vi "ReadIOValues b2g1.vi"(2 "error in":errorcluster, 3 "Output - Cluster b2g1 2":T1 {"DS-3 [bar]" format="%#.2g"; "TS-6 [°C]" format="%#.2g"; "GZ-1 [dl]" format="%.0g"; "TS-5 [°C]" format="%#.2g"; "pHS-1 [pH]" format="%.2g"; "TS-4 [°C]" format="%#.2g"; "FS-2 [l]" format="%.2g"; "FS-1 [l]" format="%.2g"; "DS-1 [bar]" format="%#.2g"; "DFS-1 [l/min]" format="%#.2g"; "FS-3 [l]" format="%.2g"; "DFS-1 [dl]" format="%.0g"}) -> (0 "error out":errorcluster, 1 "Output - Cluster b2g1":T1 {"DS-3 [bar]" format="%#.2g"; "TS-6 [°C]" format="%#.2g"; "GZ-1 [dl]" format="%.0g"; "TS-5 [°C]" format="%#.2g"; "pHS-1 [pH]" format="%.2g"; "TS-4 [°C]" format="%#.2g"; "FS-2 [l]" format="%.2g"; "FS-1 [l]" format="%.2g"; "DS-1 [bar]" format="%#.2g"; "DFS-1 [l/min]" format="%#.2g"; "FS-3 [l]" format="%.2g"; "DFS-1 [dl]" format="%.0g"})   [LabVIEW 2011]
uses:
  <vilib>/functionblocks/Counter/Count Up/Count Up.vi
  <vilib>/functionblocks/NI_FunctionBlock Libraries.lvlib
  <vilib>/functionblocks/FB Core/FB Core.xnode
  Output - Cluster b2g1.ctl
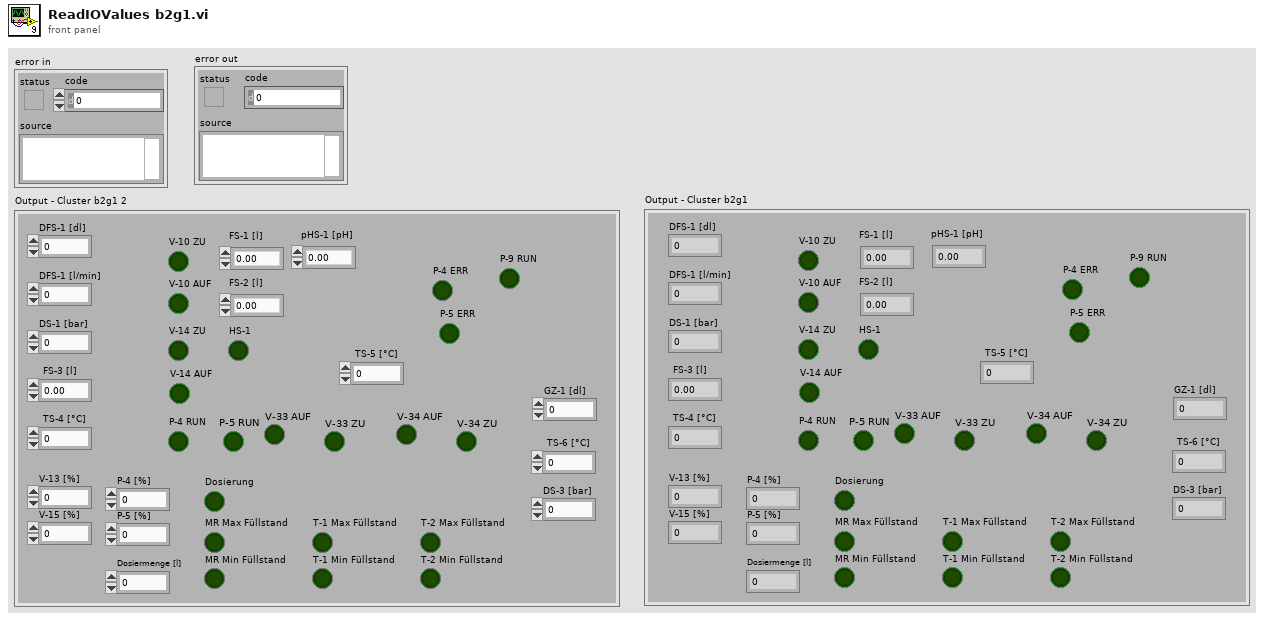
[diagram p1: front panel]
types:
  T1 = typedef "Output - Cluster b2g1.ctl" = cluster{"DFS-1 [dl]":u64, "FS-3 [l]":dbl, "DFS-1 [l/min]":dbl, "DS-1 [bar]":dbl, "V-10 ZU":bool, "V-14 ZU":bool, "FS-1 [l]":dbl, "FS-2 [l]":dbl, "TS-4 [°C]":dbl, "HS-1":bool, "V-13 [%]":u8, "V-15 [%]":u8, "P-4 [%]":u8, "P-5 [%]":u8, "Dosierung":bool, "MR Max Füllstand":bool, "MR Min Füllstand":bool, "Dosiermenge [l]":sgl, "V-14 AUF":bool, "V-10 AUF":bool, "T-1 Max Füllstand":bool, "T-1 Min Füllstand":bool, "T-2 Max Füllstand":bool, "T-2 Min Füllstand":bool, "pHS-1 [pH]":dbl, "P-4 RUN":bool, "P-5 RUN ":bool, "V-33 AUF":bool, "V-33 ZU":bool, "V-34 AUF":bool, "V-34 ZU":bool, "P-4 ERR":bool, "P-5 ERR":bool, "TS-5 [°C]":dbl, "GZ-1 [dl]":u64, "TS-6 [°C]":dbl, "DS-3 [bar]":dbl, "P-9 RUN":bool}
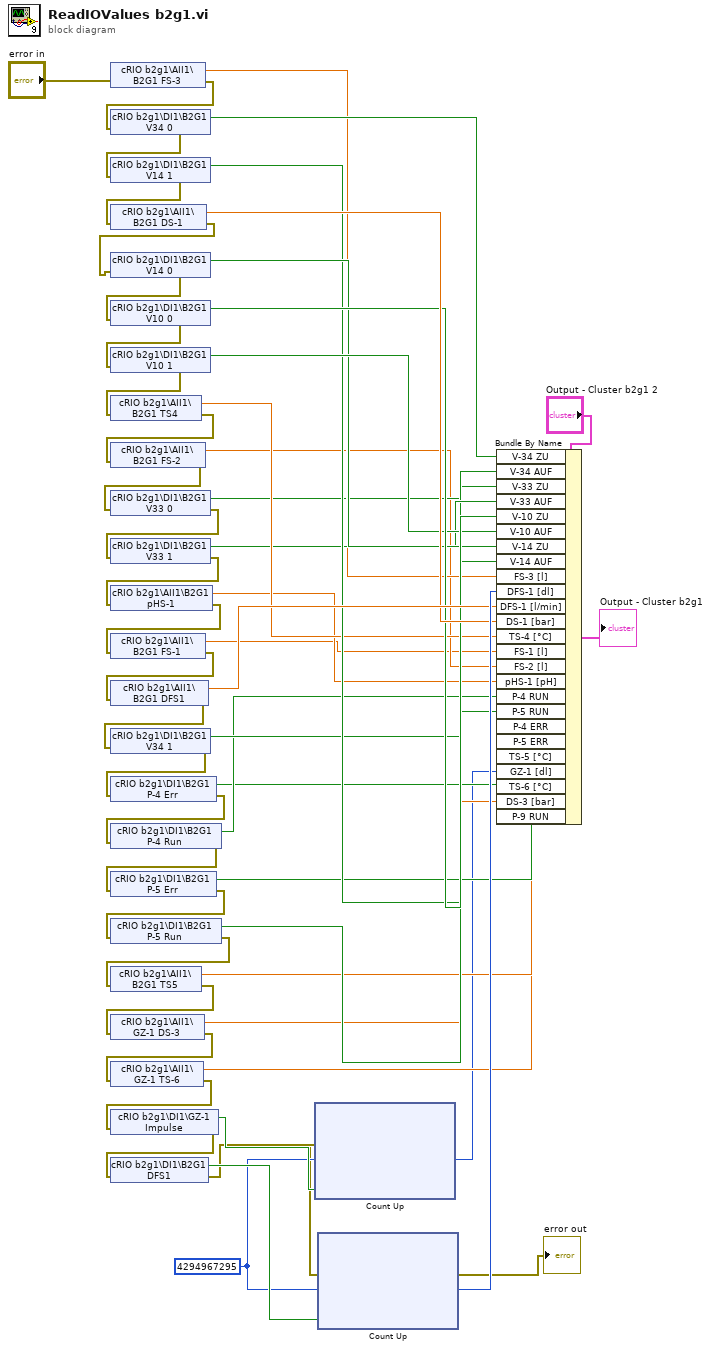
[diagram p0: block diagram]
diagram:
  w37 = u32 4294967295 ("preset value")
  n1 = shared-variable "cRIO b2g1\\AII1\\B2G1 FS-3"(error in="error in") -> (w19:dbl, error out=w26:errorcluster)
  n2 = shared-variable "cRIO b2g1\\DI1\\B2G1 V34 0"(error in=w26) -> (w45:bool, error out=w25:errorcluster)
  n3 = shared-variable "cRIO b2g1\\DI1\\B2G1 V14 1"(error in=w25) -> (w49:bool, error out=w24:errorcluster)
  n4 = shared-variable "cRIO b2g1\\AII1\\B2G1 DS-1"(error in=w24) -> (w53:dbl, error out=w23:errorcluster)
  n5 = shared-variable "cRIO b2g1\\DI1\\B2G1 V14 0"(error in=w23) -> (w50:bool, error out=w22:errorcluster)
  n6 = shared-variable "cRIO b2g1\\DI1\\B2G1 V10 0"(error in=w22) -> (w52:bool, error out=w21:errorcluster)
  n7 = shared-variable "cRIO b2g1\\DI1\\B2G1 V10 1"(error in=w21) -> (w51:bool, error out=w20:errorcluster)
  n8 = shared-variable "cRIO b2g1\\AII1\\B2G1 TS4"(error in=w20) -> (w48:dbl, error out=w17:errorcluster)
  n9 = shared-variable "cRIO b2g1\\AII1\\B2G1 FS-2"(error in=w17) -> (w2:dbl, error out=w16:errorcluster)
  n10 = shared-variable "cRIO b2g1\\DI1\\B2G1 V33 0"(error in=w16) -> (w18:bool, error out=w15:errorcluster)
  n11 = shared-variable "cRIO b2g1\\DI1\\B2G1 V33 1"(error in=w15) -> (w46:bool, error out=w14:errorcluster)
  n12 = shared-variable "cRIO b2g1\\AII1\\B2G1 pHS-1"(error in=w14) -> (w47:dbl, error out=w13:errorcluster)
  n13 = shared-variable "cRIO b2g1\\AII1\\B2G1 FS-1"(error in=w13) -> (w1:dbl, error out=w12:errorcluster)
  n14 = shared-variable "cRIO b2g1\\AII1\\B2G1 DFS1"(error in=w12) -> (w54:dbl, error out=w11:errorcluster)
  n15 = shared-variable "cRIO b2g1\\DI1\\B2G1 V34 1"(error in=w11) -> (w44:bool, error out=w10:errorcluster)
  n16 = shared-variable "cRIO b2g1\\DI1\\B2G1 P-4 Err"(error in=w10) -> (w41:bool, error out=w9:errorcluster)
  n17 = shared-variable "cRIO b2g1\\DI1\\B2G1 P-4 Run"(error in=w9) -> (w43:bool, error out=w8:errorcluster)
  n18 = shared-variable "cRIO b2g1\\DI1\\B2G1 P-5 Err"(error in=w8) -> (w40:bool, error out=w7:errorcluster)
  n19 = shared-variable "cRIO b2g1\\DI1\\B2G1 P-5 Run"(error in=w7) -> (w42:bool, error out=w6:errorcluster)
  n20 = shared-variable "cRIO b2g1\\AII1\\B2G1 TS5"(error in=w6) -> (w39:dbl, error out=w3:errorcluster)
  n21 = shared-variable "cRIO b2g1\\AII1\\GZ-1 DS-3"(error in=w3) -> (w35:dbl, error out=w5:errorcluster)
  n22 = shared-variable "cRIO b2g1\\AII1\\GZ-1 TS-6"(error in=w5) -> (w36:dbl, error out=w4:errorcluster)
  n23 = shared-variable "cRIO b2g1\\DI1\\GZ-1 Impulse"(error in=w4) -> (w38:bool, error out=w29:errorcluster)
  n24 = shared-variable "cRIO b2g1\\DI1\\B2G1 DFS1"(error in=w29) -> (w56:bool, error out=w28:errorcluster)
  n25 = xnode "Count Up"("error in"=w28, "preset value"=w37, "count up"=w38) -> ("error out"=w27:errorcluster, "counter value"=w34:u32)  [unwired: 1 in, 1 out]
  n26 = xnode "Count Up"("error in"=w27, "preset value"=w37, "count up"=w56) -> ("error out"=→"error out":errorcluster, "counter value"=w55:u32)  [unwired: 1 in, 1 out]
  n27 = Bundle By Name(cluster="Output - Cluster b2g1 2", "V-34 ZU"=w45, "V-34 AUF"=w44, "V-33 ZU"=w18, "V-33 AUF"=w46, "V-10 ZU"=w52, "V-10 AUF"=w51, "V-14 ZU"=w50, "V-14 AUF"=w49, "FS-3 [l]"=w19, "DFS-1 [dl]"=w55, "DFS-1 [l/min]"=w54, "DS-1 [bar]"=w53, "TS-4 [°C]"=w48, "FS-1 [l]"=w1, "FS-2 [l]"=w2, "pHS-1 [pH]"=w47, "P-4 RUN"=w43, "P-5 RUN"=w42, "P-4 ERR"=w41, "P-5 ERR"=w40, "TS-5 [°C]"=w39, "GZ-1 [dl]"=w34, "TS-6 [°C]"=w36, "DS-3 [bar]"=w35) -> (→"Output - Cluster b2g1":T1)  [unwired: 1 in]
